vi "importer_@.vi"() -> ()   [LabVIEW 2016]
uses:
  Experiment/Experiment.lvclass
panel:
  out "Error":bool
  in  "Scanning":bool
  in  "Remote Stop":bool
  in  "Analog Signals":bool=TRUE
  in  "Ball Motion":bool=TRUE
  in  "Video":bool=TRUE
  in  "stop":bool
  in  "Tab Control":enum32{"Session", "Scan"}(tab)
  in  "Session Start":bool
  in  "Session Cluster":T1
  in  "Scan Stop":bool
  in  "Scan Start":bool
  in  "Scan Cluster":T2
  out "error out":errorcluster
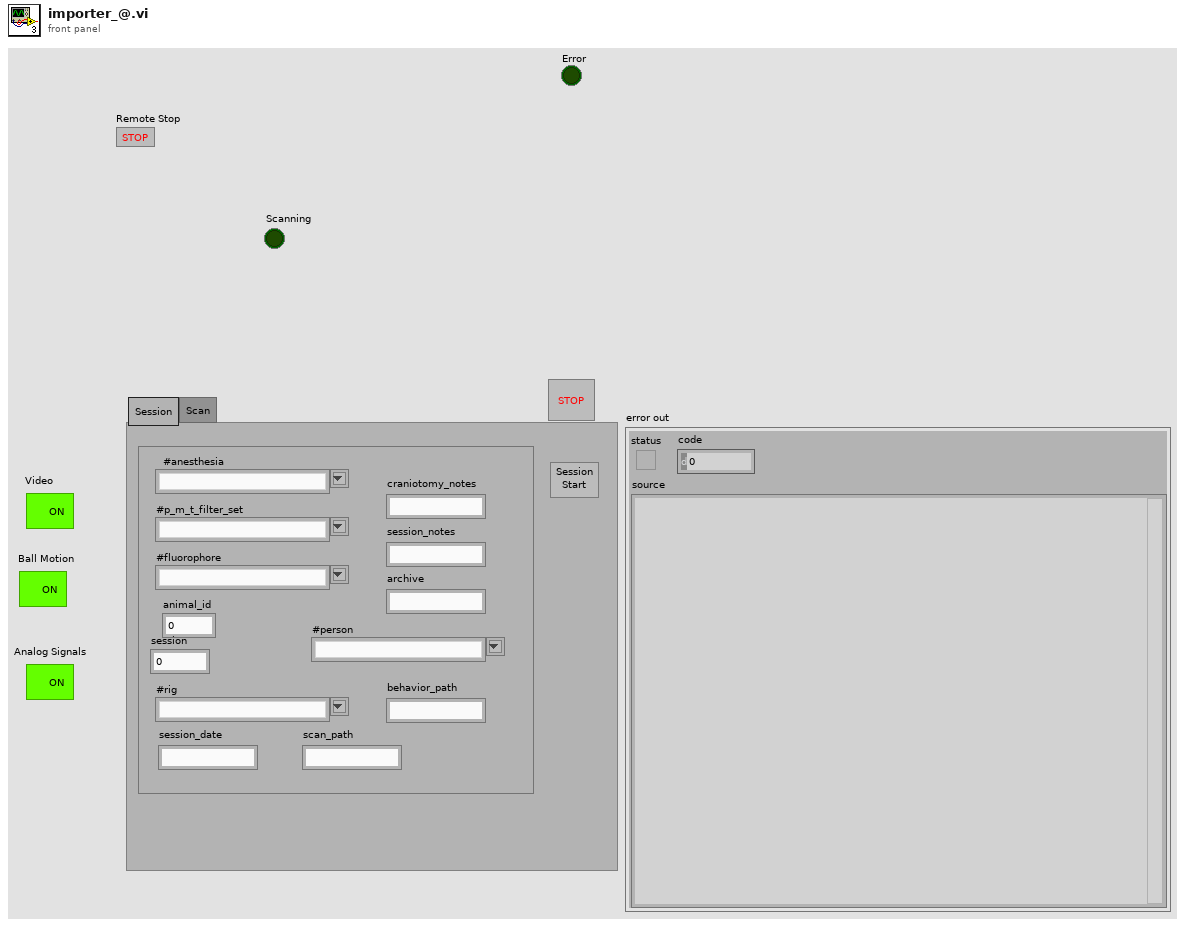
[diagram p1: front panel]
types:
  T1 = cluster{"#p_m_t_filter_set":string, "#anesthesia":string, "#fluorophore":string, "animal_id":dbl, "#rig":string, "session":dbl, "session_date":string, "#person":string, "scan_path":string, "behavior_path":string, "craniotomy_notes":string, "session_notes":string, "archive":string}
  T2 = cluster{"#brain_area":string, "#software":string, "#lens":string, "filename":string, "depth":dbl, "scan_notes":string, "site_number":dbl, "scan_idx":dbl, "animal_id":dbl, "session":dbl}
  T3 = enum8{"Enabled", "Disabled", "Disabled and Grayed Out"}
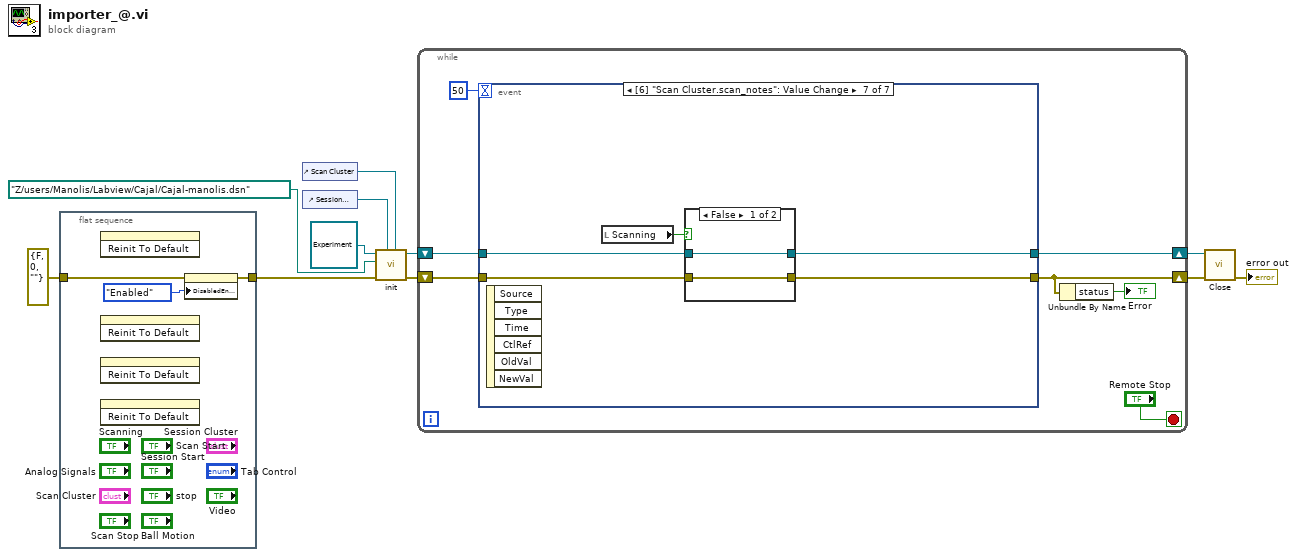
[diagram p0: block diagram]
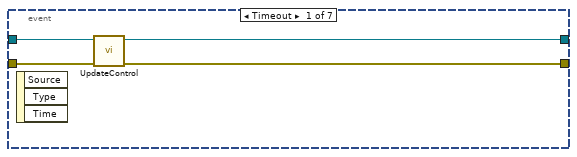
[diagram p2: hidden frame]
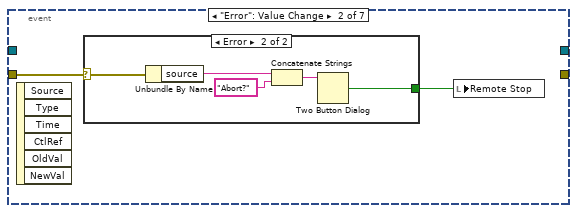
[diagram p3: hidden frame]
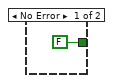
[diagram p4: hidden frame]
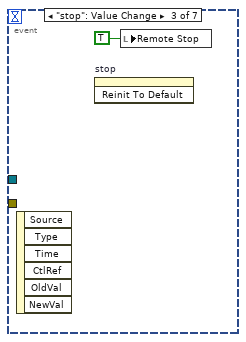
[diagram p5: hidden frame]
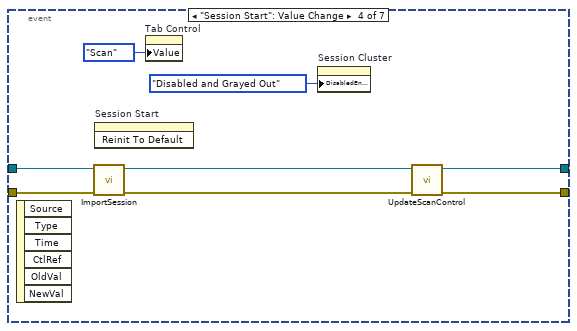
[diagram p6: hidden frame]
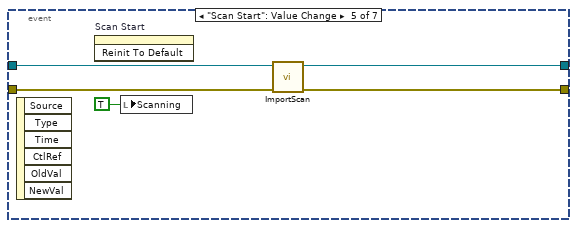
[diagram p7: hidden frame]
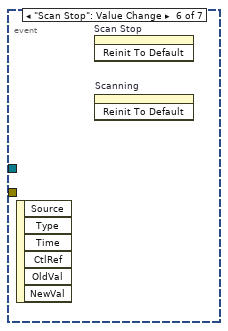
[diagram p8: hidden frame]
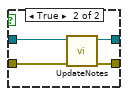
[diagram p9: hidden frame]
diagram:
  n1 = flat-sequence {
    tunnel: errorcluster {"status"=FALSE, "code"=0, "source"=""} ("error in (no error)") -> [w13]
    tunnel: [w12] -> w2
    frame #0 {
      n2 = invoke on="Remote Stop" class="Bool (strict)" method="Reinit To Default"() -> ()  [unwired: 3 in, 3 out]
      n3 = invoke on="Scanning" class="Bool (strict)" method="Reinit To Default"() -> ()  [unwired: 3 in, 3 out]
      n4 = invoke on="stop" class="Bool (strict)" method="Reinit To Default"() -> ()  [unwired: 3 in, 3 out]
      n5 = invoke on="error out" class="Clust (strict)" method="Reinit To Default"() -> ()  [unwired: 3 in, 3 out]
      n6 = property on="Session Cluster" class="Clust (strict)"(error in=w13, "DisabledEnum"=T3."Enabled" ("Disabled")) -> (error out=w12:errorcluster)  [unwired: 1 in, 1 out]
    }
  }
  n7 = control-ref of="Scan Cluster"() -> (w4:refnum<vi>)
  n8 = control-ref of="Session Cluster"() -> (w5:refnum<vi>)
  n9 = call-dynamic "init.vi"("Scan control"=w4, "Session control"=w5, "error in (no error)"=w2, "Session - Pipeline"=path "Z:/users/Manolis/Labview/Cajal/Cajal-manolis.dsn", "Experiment in"=refnum<class "Experiment.lvclass"> refnum ("Experiment.lvclass")) -> ("error out"=w9:errorcluster, "Experiment out"=w8:refnum<class "Experiment.lvclass">)  [unwired: 5 in]
  n10 = while {
    shift-right: [w16] -> w7
    shift-left: w9 -> [w21]
    shift-right: [w19] -> w6
    shift-left: w8 -> [w18]
    stop <- "Remote Stop" stop-if-true
    n11 = event shown="[6] \"Scan Cluster.scan_notes\": Value Change" {
      selector: _ -> [_ _ _ _ _ _ _]
      dyn-events: _ -> [_ _ _ _ _ _ _]
      timeout: 50 -> [_ _ _ _ _ _ _]
      tunnel: w21 -> [w24 w27 _ w41 w46 _ w50]
      tunnel: [w22 _ _ w35 w45 _ w48] -> w16
      tunnel: w18 -> [w25 _ _ w42 w47 _ w51]
      tunnel: [w23 _ _ w36 w44 _ w49] -> w19
      event Timeout {
        n12 = event-data() -> ()  [unwired: 1 in, 3 out]
        n13 = call-dynamic "UpdateControl.vi"("error in (no error)"=w24, "Experiment in"=w25) -> ("error out"=w22:errorcluster, "Experiment out"=w23:refnum<class "Experiment.lvclass">)  [unwired: 8 in]
      }
      event "Error": Value Change {
        n14 = event-data() -> ()  [unwired: 1 in, 6 out]
        n15 = case shown="Error" w27 {
          selector: w27 -> [_ w32]
          tunnel: [FALSE ("T button?") w33] -> w26
          frame No Error {
          }
          frame Error {
            n16 = Unbundle By Name(w32) -> ("source"=w31:string)
            n17 = Concatenate Strings(w31, "Abort?" ("message")) -> (w29:string)
            n18 = Two Button Dialog(message=w29) -> (T button?=w33:bool)  [unwired: 2 in]
          }
        }
        n19 = local write "Remote Stop"(w26) -> ()
      }
      event "stop": Value Change {
        n20 = event-data() -> ()  [unwired: 1 in, 6 out]
        n21 = invoke on="stop" class="Bool (strict)" method="Reinit To Default"() -> ()  [unwired: 3 in, 3 out]
        n22 = local write "Remote Stop"(TRUE ("Remote Stop")) -> ()
      }
      event "Session Start": Value Change {
        n23 = event-data() -> ()  [unwired: 1 in, 6 out]
        n24 = call-dynamic "ImportSession.vi"("error in (no error)"=w41, "Experiment in"=w42) -> ("error out"=w37:errorcluster, "Experiment out"=w38:refnum<class "Experiment.lvclass">)  [unwired: 8 in]
        n25 = invoke on="Session Start" class="Bool (strict)" method="Reinit To Default"() -> ()  [unwired: 3 in, 3 out]
        n26 = property on="Tab Control" class="TabCtl (strict)"("Value"=enum32{"Session", "Scan"}."Scan" ("Tab Control")) -> ()  [unwired: 2 in, 2 out]
        n27 = property on="Session Cluster" class="Clust (strict)"("DisabledEnum"=T3."Disabled and Grayed Out" ("Disabled")) -> ()  [unwired: 2 in, 2 out]
        n28 = call-dynamic "UpdateScanControl.vi"("error in (no error)"=w37, "Experiment in"=w38) -> ("error out"=w35:errorcluster, "Experiment out"=w36:refnum<class "Experiment.lvclass">)  [unwired: 8 in]
      }
      event "Scan Start": Value Change {
        n29 = event-data() -> ()  [unwired: 1 in, 6 out]
        n30 = invoke on="Scan Start" class="Bool (strict)" method="Reinit To Default"() -> ()  [unwired: 3 in, 3 out]
        n31 = local write "Scanning"(TRUE ("Scanning")) -> ()
        n32 = call-dynamic "ImportScan.vi"("error in (no error)"=w46, "Experiment in"=w47) -> ("error out"=w45:errorcluster, "Experiment out"=w44:refnum<class "Experiment.lvclass">)  [unwired: 8 in]
      }
      event "Scan Stop": Value Change {
        n33 = event-data() -> ()  [unwired: 1 in, 6 out]
        n34 = invoke on="Scan Stop" class="Bool (strict)" method="Reinit To Default"() -> ()  [unwired: 3 in, 3 out]
        n35 = invoke on="Scanning" class="Bool (strict)" method="Reinit To Default"() -> ()  [unwired: 3 in, 3 out]
      }
      event "Scan Cluster.scan_notes": Value Change {
        n36 = event-data() -> ()  [unwired: 1 in, 6 out]
        n37 = local read "Scanning"() -> (w52:bool)
        n38 = case shown="False" w52 {
          tunnel: w51 -> [w54 w58]
          tunnel: w50 -> [w53 w55]
          tunnel: [w54 w57] -> w49
          tunnel: [w53 w56] -> w48
          frame False {
          }
          frame True {
            n39 = call-dynamic "UpdateNotes.vi"("error in (no error)"=w55, "Experiment in"=w58) -> ("error out"=w56:errorcluster, "Experiment out"=w57:refnum<class "Experiment.lvclass">)  [unwired: 8 in]
          }
        }
      }
    }
    n40 = Unbundle By Name(w16) -> ("status"=→"Error":bool)
  }
  n41 = call-dynamic "Close.vi"("error in (no error)"=w7, "Experiment in"=w6) -> ("error out"=→"error out":errorcluster)  [unwired: 8 in, 1 out]
